vi "Create X Rotation Matrix.vi"(11 "Theta (°)":sgl) -> (3 "Rotation X Matrix":sgl[][](array[numeric]))   [LabVIEW 2020, in "3D.lvlib"]
uses:
  Libraries/3D/3D.lvlib
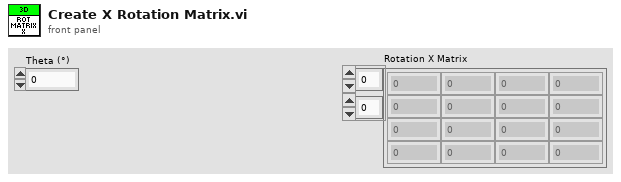
[diagram p1: front panel]
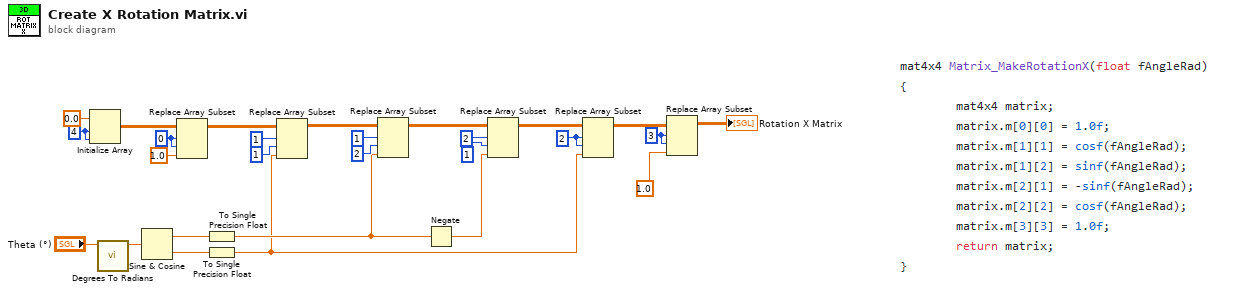
[diagram p0: block diagram]
diagram:
  w23 = 3 ("index (row)")
  w21 = 2 ("index (row)")
  w11 = 0 ("index (row)")
  w26 = 4 ("dimension size")
  n1 = Initialize Array(sgl 0.0 ("element"), w26, w26) -> (w10:sgl[][])
  n2 = call "Degrees To Radians.vi"("Angle (°)"="Theta (°)") -> ("Angle (rad)"=w1:sgl)  [unwired: 10 in]
  n3 = Sine & Cosine(0:w1) -> (1:w6:sgl, 2:w4:sgl)
  n4 = Replace Array Subset(array=w10, new element=sgl 1.0 ("new element/subarray"), index (row)=w11, index (col)=w11) -> (w12:sgl[][])
  n5 = To Single Precision Float(number=w6) -> (single precision float=w5:sgl)
  n6 = To Single Precision Float(number=w4) -> (single precision float=w3:sgl)
  n7 = Replace Array Subset(array=w12, new element=w3, index (row)=1, index (col)=1 ("disabled index (col)")) -> (w15:sgl[][])
  n8 = Replace Array Subset(array=w15, new element=w5, index (row)=1, index (col)=2 ("index (row)")) -> (w16:sgl[][])
  n9 = Negate(x=w5) -> (-x=w8:sgl)
  n10 = Replace Array Subset(array=w16, new element=w8, index (row)=2, index (col)=1 ("index (row)")) -> (w17:sgl[][])
  n11 = Replace Array Subset(array=w17, new element=w3, index (row)=w21, index (col)=w21) -> (w22:sgl[][])
  n12 = Replace Array Subset(array=w22, new element=sgl 1.0 ("new element/subarray"), index (row)=w23, index (col)=w23) -> (→"Rotation X Matrix":sgl[][])
